vi "manual test UI.vi"(8 "error in (no error)":errorcluster caption="Fehler (Eingang, kein Fehler)", 11 "Surge Eingang":refnum<class "Surge.lvclass"> caption="DNL_LabVIEW Object in") -> (0 "error out":errorcluster caption="Fehler (Ausgang)", 1 "parameters":string[][](table), 2 "Parameters":u32[](array[numeric]), 3 "Surge Ausgang":refnum<class "Surge.lvclass"> caption="DNL_LabVIEW Object out", 5 "abbrechen":bool)   [LabVIEW 2013, in "Surge.lvclass"]
uses:
  Surge.lvclass
panel:
  in  "270°":bool
  in  "0°":bool
  in  "90°":bool
  in  "Spannung in V":u32=200 min=200 max=4200
  in  "Abbrechen":bool
  in  "OK":bool
  in  "N-PE":bool
  in  "PE-L1":bool
  in  "N-L1":bool
  in  "PE-N":bool
  in  "L1-N":bool
  in  "L1-PE":bool
  in  "Pause in s":u32=10 min=10 max=999
  in  "Wiederholungen":u32=1 min=1 max=999
  # "Kopplung"
  # "Phaseneintritt"
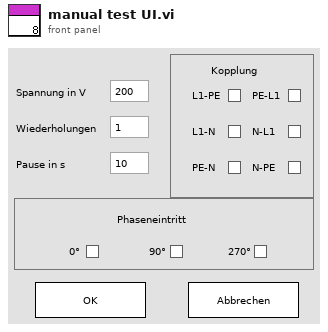
[diagram p1: front panel]
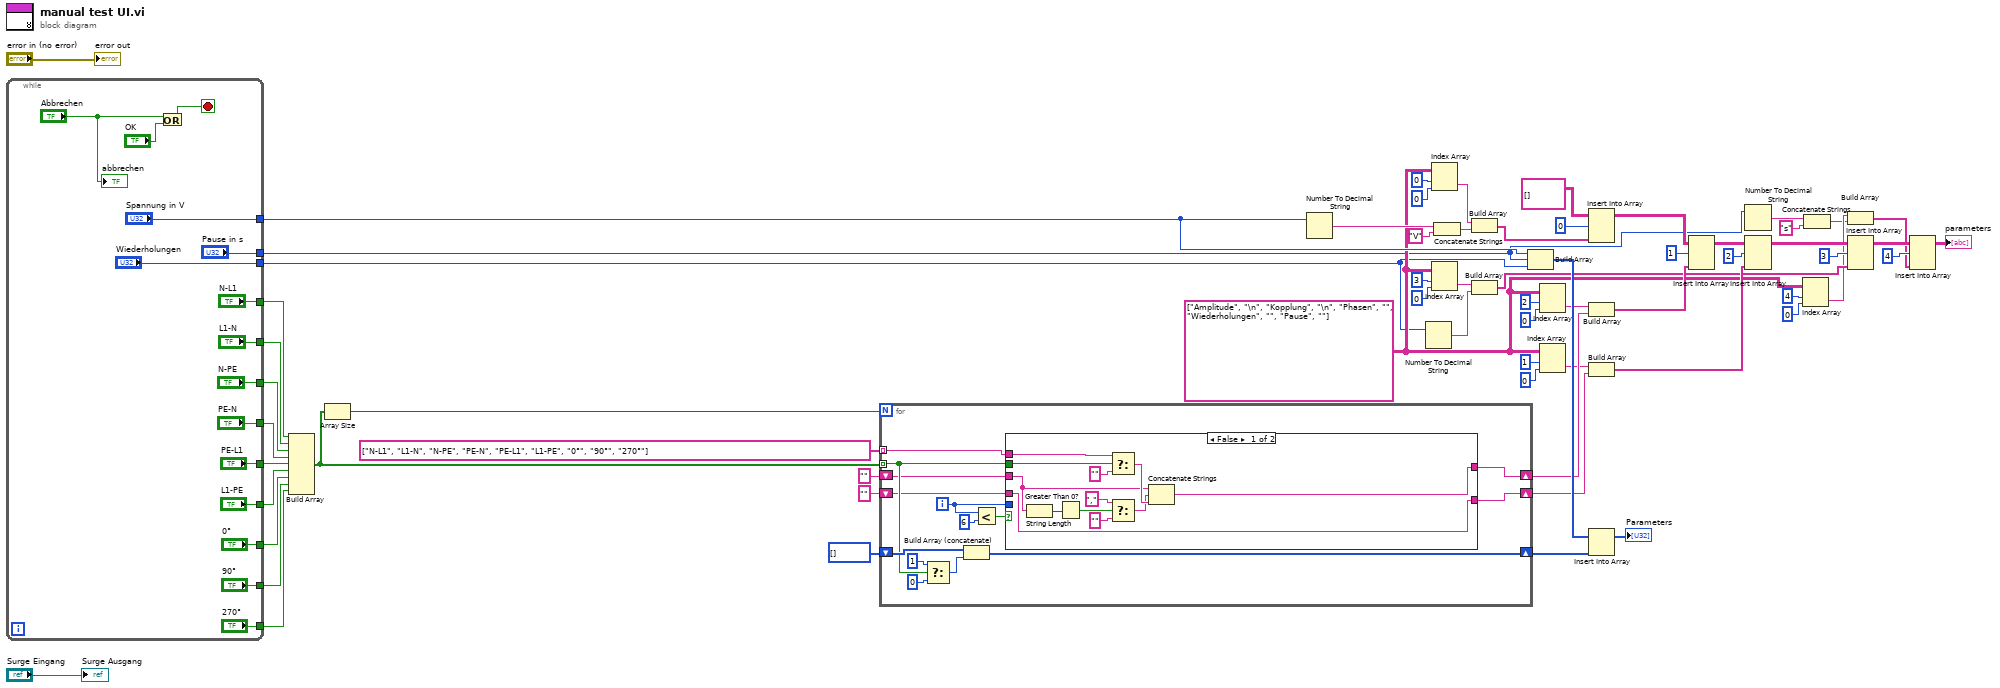
[diagram p0: block diagram]
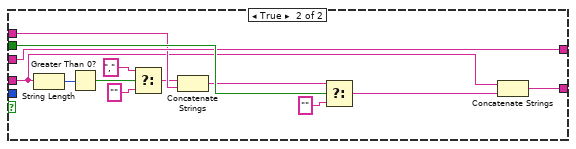
[diagram p2: hidden frame]
diagram:
  w8 = string[][] [["Amplitude", "\n"], ["Kopplung", "\n"], ["Phasen", ""], ["Wiederholungen", ""], ["Pause", ""]]
  n1 = while {
    tunnel: ["N-L1"] -> w63
    tunnel: ["L1-N"] -> w62
    tunnel: ["N-PE"] -> w61
    tunnel: ["PE-N"] -> w60
    tunnel: ["PE-L1"] -> w59
    tunnel: ["L1-PE"] -> w58
    tunnel: ["Pause in s"] -> w1
    tunnel: ["Wiederholungen"] -> w2
    tunnel: ["Spannung in V"] -> w35
    tunnel: ["0°"] -> w48
    tunnel: ["90°"] -> w47
    tunnel: ["270°"] -> w46
    stop <- w70 stop-if-true
    n2 = Or(x="Abbrechen", y="OK") -> (x .or. y?=w70:bool)
    "abbrechen" <- "Abbrechen"
  }
  n3 = Build Array(w63, w62, w61, w60, w59, w58, w48, w47, w46) -> (w54:bool[])
  n4 = Array Size(array=w54) -> (size(s)=w55:i32)
  n5 = for {
    N: w55 -> [_]
    tunnel: w54 -> [w88] mode=indexing
    shift-right: [w89] -> w52
    shift-left: u32[] [] -> [w93]
    tunnel: string[] ["N-L1", "L1-N", "N-PE", "PE-N", "PE-L1", "L1-PE", "0°", "90°", "270°"] -> [w87] mode=indexing
    shift-right: [w81] -> w28
    shift-left: "" -> [w86]
    shift-right: [w83] -> w30
    shift-left: "" -> [w82]
    i -> [w80]
    n6 = Select(t=u32 1, s=w88, f=u32 0) -> (s? t:f=w92:u32)
    n7 = Build Array (concatenate)(w93, w92) -> (w89:u32[])
    n8 = Less?(x=w80, y=6) -> (x < y?=w84:bool)
    n9 = case shown="False" w84 {
      tunnel: w88 -> [w101 w118]
      tunnel: w87 -> [w100 w114]
      tunnel: [w105 w116] -> w81
      tunnel: w86 -> [w105 w108]
      tunnel: [w102 w115] -> w83
      tunnel: w82 -> [w97 w115]
      tunnel: w80 -> [_ _]
      frame False {
        n10 = String Length(string=w97) -> (length=w98:i32)
        n11 = Greater Than 0?(x=w98) -> (x > 0?=w96:bool)
        n12 = Select(t=w100, s=w101, f="") -> (s? t:f=w103:string)
        n13 = Select(t="," ("string"), s=w96, f="") -> (s? t:f=w94:string)
        n14 = Concatenate Strings(w97, w94, w103) -> (w102:string)
      }
      frame True {
        n15 = String Length(string=w108) -> (length=w107:i32)
        n16 = Greater Than 0?(x=w107) -> (x > 0?=w106:bool)
        n17 = Select(t="," ("string"), s=w106, f="") -> (s? t:f=w109:string)
        n18 = Concatenate Strings(w109, w114) -> (w113:string)
        n19 = Select(t=w113, s=w118, f="") -> (s? t:f=w112:string)
        n20 = Concatenate Strings(w108, w112) -> (w116:string)
      }
    }
  }
  n21 = Number To Decimal String(number=w35) -> (decimal integer string=w20:string)  [unwired: 1 in]
  n22 = Number To Decimal String(number=w2) -> (decimal integer string=w14:string)  [unwired: 1 in]
  n23 = Index Array(array=w8, index (row)=0, index (col)=0 ("disabled index (col)")) -> (element=w27:string)
  n24 = Index Array(array=w8, index (row)=3, index (col)=0 ("disabled index (col)")) -> (element=w21:string)
  n25 = Concatenate Strings(w20, "V" ("string")) -> (w18:string)
  n26 = Build Array(w27, w18) -> (w32:string[])
  n27 = Build Array(w21, w14) -> (w16:string[])
  n28 = Build Array(w35, w1, w2) -> (w56:u32[])
  n29 = Index Array(array=w8, index (row)=2, index (col)=0 ("disabled index (col)")) -> (element=w31:string)
  n30 = Index Array(array=w8, index (row)=1, index (col)=0 ("disabled index (col)")) -> (element=w29:string)
  n31 = Insert Into Array(array=string[][] [], index (row)=0, new element=w32) -> (w25:string[][])  [unwired: 1 in]
  n32 = Build Array(w31, w30) -> (w37:string[])
  n33 = Build Array(w29, w28) -> (w41:string[])
  n34 = Insert Into Array(array=w56, new element=w52) -> (→"Parameters":u32[])  [unwired: 1 in]
  n35 = Insert Into Array(array=w25, index (row)=1, new element=w37) -> (w24:string[][])  [unwired: 1 in]
  n36 = Number To Decimal String(number=w1) -> (decimal integer string=w6:string)  [unwired: 1 in]
  n37 = Insert Into Array(array=w24, index (row)=2, new element=w41) -> (w17:string[][])  [unwired: 1 in]
  n38 = Index Array(array=w8, index (row)=4, index (col)=0 ("disabled index (col)")) -> (element=w7:string)
  n39 = Concatenate Strings(w6, "s" ("string")) -> (w4:string)
  n40 = Build Array(w7, w4) -> (w11:string[])
  n41 = Insert Into Array(array=w17, index (row)=3, new element=w16) -> (w12:string[][])  [unwired: 1 in]
  n42 = Insert Into Array(array=w12, index (row)=4, new element=w11) -> (→"parameters":string[][])  [unwired: 1 in]
  "error out" <- "error in (no error)"
  "Surge Ausgang" <- "Surge Eingang"
